vi "Add Correction.vi"(8 "error in (no error)":errorcluster, 9 "Assembly Type":string, 10 "XYZTheta":dbl[](array[numeric]), 11 "Carrier Tray in":refnum<class "Assembly Tray.lvclass">) -> (0 "error out":errorcluster, 2 "XYZTheta Out":dbl[](array[numeric]), 3 "Carrier Tray out":refnum<class "Assembly Tray.lvclass">)   [LabVIEW 2021, in "Assembly Tray.lvclass"]
uses:
  Assembly Tray.lvclass
  C:/Users/HEP/Documents/GitHub/Gantry/UCSB-Gantry-HEP-main/Classes/Workspace/Fixture.lvclass
  Fixture.lvclass/Fixture.ctl
  Read Fixture ID.vi
  Read Position.vi
  Routine/Pick and Place/Pick and Place.lvclass
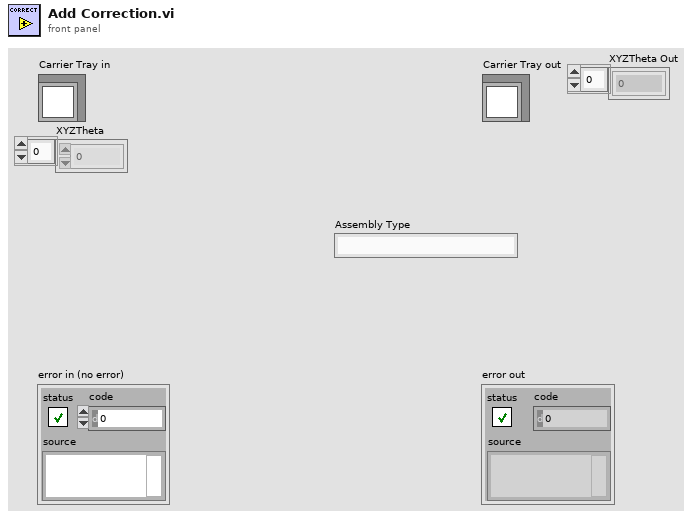
[diagram p1: front panel]
types:
  T1 = typedef "File Paths.ctl" = cluster{"Glue Pattern Folder":path, "Carrier Tray Folder":path, "Pick Up Tool Fixture Folder":path, "Components Folder":path, "Bellows Tool Offset.txt":path, "Pick Up Tool Offset.txt":path, "Dispense Tip Offset.txt":path, "Log Files":path, "Gantry Assembly Map.txt":path, "Syringe and offset map.txt":path, "Controllers Folder":path, "Local dbase config":path}
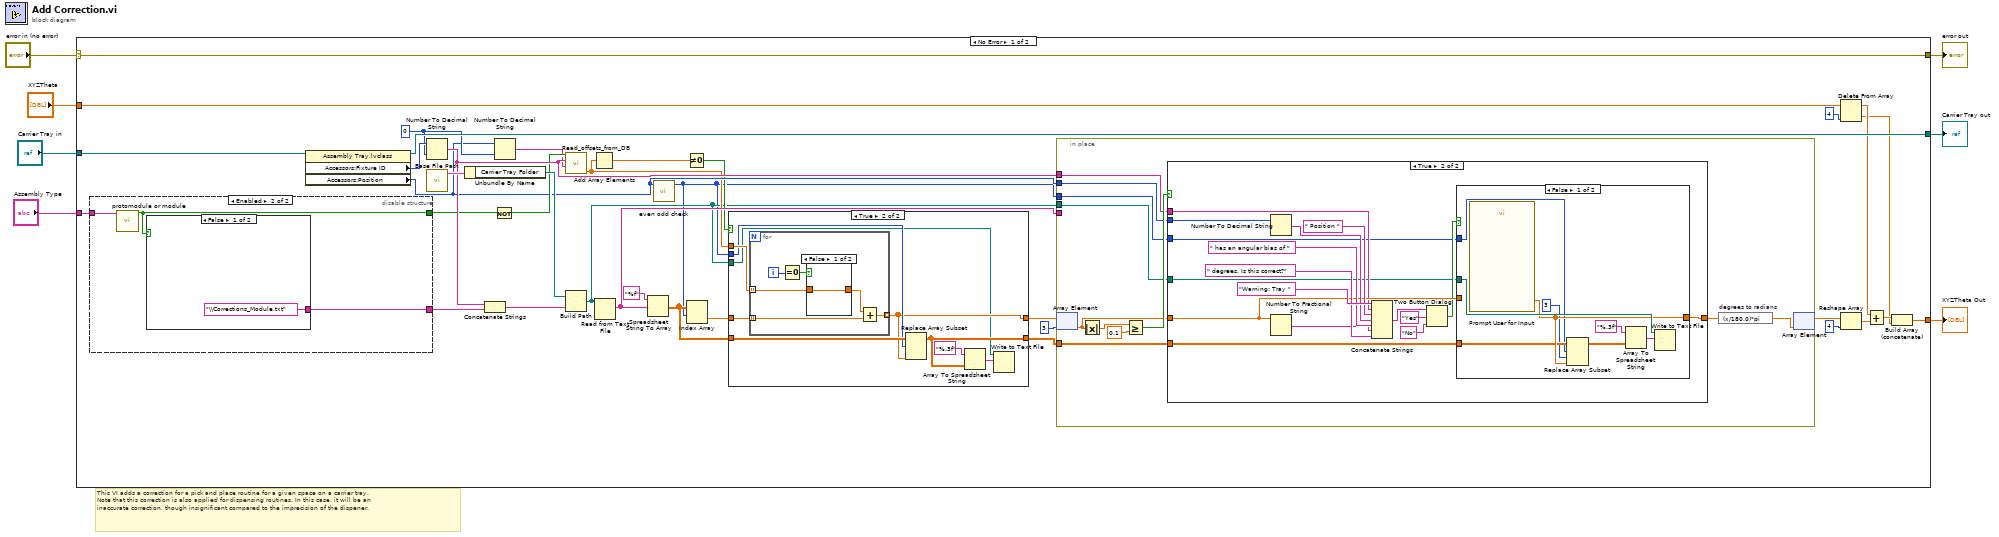
[diagram p0: block diagram]
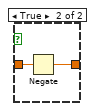
[diagram p3: hidden frame]
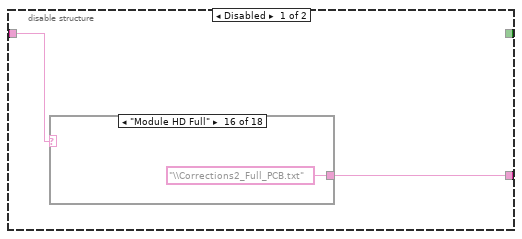
[diagram p6: hidden frame]
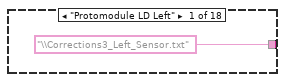
[diagram p7: hidden frame]
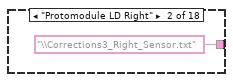
[diagram p8: hidden frame]
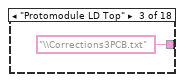
[diagram p9: hidden frame]
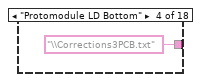
[diagram p10: hidden frame]
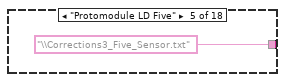
[diagram p11: hidden frame]
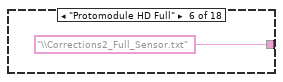
[diagram p12: hidden frame]
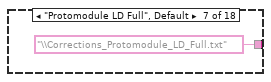
[diagram p13: hidden frame]
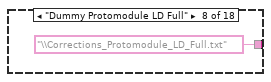
[diagram p14: hidden frame]
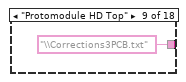
[diagram p15: hidden frame]
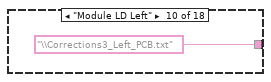
[diagram p16: hidden frame]
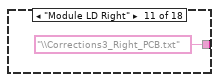
[diagram p17: hidden frame]
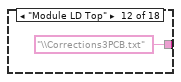
[diagram p18: hidden frame]
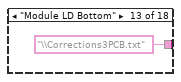
[diagram p19: hidden frame]
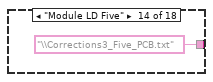
[diagram p20: hidden frame]
diagram:
  # "This VI adds a correction for a pick and place routine for a given space on a carrier tray.\nNote that this correction is also applied for dispensing routines. In this case, it will be an\ninaccurate correction, though insignificant compared to the imprecision of the dispener."
  n1 = case shown="No Error" "error in (no error)" {
    selector: "error in (no error)" -> [w43 w129]
    tunnel: [w43 w129] -> w6
    tunnel: [w34 w128] -> w4
    tunnel: "Carrier Tray in" -> [w35 w128]
    tunnel: "XYZTheta" -> [w31 w127]
    tunnel: [w26 w127] -> w2
    tunnel: "Assembly Type" -> [w32 _]
    frame No Error {
      w19 = i16 0 ("width (-)")
      n2 = disable-structure shown="Enabled" {
        disable-tunnel: [w103 w124] -> w40
        disable-tunnel: w32 -> [w102 w123]
        disable-tunnel: [_ w122] -> w21
        frame Disabled {
          n3 = case shown="\"Module HD Full\"" w102 {
            tunnel: ["\\Corrections3_Left_Sensor.txt" ("name or relative path") "\\Corrections3_Right_Sensor.txt" ("name or relative path") "\\Corrections3PCB.txt" ("name or relative path") "\\Corrections3PCB.txt" ("name or relative path") "\\Corrections3_Five_Sensor.txt" ("name or relative path") "\\Corrections2_Full_Sensor.txt" ("name or relative path") "\\Corrections_Protomodule_LD_Full.txt" ("name or relative path") "\\Corrections_Protomodule_LD_Full.txt" ("name or relative path") "\\Corrections3PCB.txt" ("name or relative path") "\\Corrections3_Left_PCB.txt" ("name or relative path") "\\Corrections3_Right_PCB.txt" ("name or relative path") "\\Corrections3PCB.txt" ("name or relative path") "\\Corrections3PCB.txt" ("name or relative path") "\\Corrections3_Five_PCB.txt" ("name or relative path") "\\Corrections2_Full_PCB.txt" ("name or relative path") "\\Corrections2_Full_PCB.txt" ("name or relative path") "\\Corrections_Module_LD_Full.txt" ("name or relative path") "\\Corrections_Module_LD_Full.txt" ("name or relative path")] -> w103
            frame "Protomodule LD Left" {
            }
            frame "Protomodule LD Right" {
            }
            frame "Protomodule LD Top" {
            }
            frame "Protomodule LD Bottom" {
            }
            frame "Protomodule LD Five" {
            }
            frame "Protomodule HD Full" {
            }
            frame "Protomodule LD Full", Default {
            }
            frame "Dummy Protomodule LD Full" {
            }
            frame "Protomodule HD Top" {
            }
            frame "Module LD Left" {
            }
            frame "Module LD Right" {
            }
            frame "Module LD Top" {
            }
            frame "Module LD Bottom" {
            }
            frame "Module LD Five" {
            }
            frame "Module HD Top" {
            }
            frame "Module HD Full" {
            }
            frame "Module LD Full" {
            }
            frame "Dummy Module LD Full" {
            }
          }
        }
        frame Enabled {
          n4 = call "protomodule or module.vi"("assembly type"=w123) -> ("protomodule? (T)"=w122:bool)  [unwired: 10 in]
          n5 = case shown="False" w122 {
            tunnel: ["\\Corrections_Module.txt" ("name or relative path") "\\Corrections_Protomodule.txt" ("name or relative path")] -> w124
            frame False {
            }
            frame True {
            }
          }
        }
      }
      n6 = property class="Assembly Tray.lvclass"(reference=w35) -> (reference out=w34:refnum<class "Assembly Tray.lvclass">, "Accessors:Fixture ID"=w33:i32, "Accessors:Position"=w18:i32)  [unwired: 1 in, 1 out]
      n7 = Number To Decimal String(number=w33, width (-)=w19) -> (decimal integer string=w22:string)
      n8 = call "Base File Path.vi"() -> ("Paths Out"=w42:T1)  [unwired: 11 in]
      n9 = Unbundle By Name(w42) -> ("Carrier Tray Folder"=w41:path)
      n10 = Concatenate Strings(w22, w40) -> (w39:string)
      n11 = Not(x=w21) -> (.not. x?=w20:bool)
      n12 = Number To Decimal String(number=w18, width (-)=w19) -> (decimal integer string=w17:string)
      n13 = call "Read_offsets_from_DB.vi"("PUT position"=w17, "Assembly Tray ID"=w22, "Module?"=w20) -> ("Bias to add"=w14:dbl[])  [unwired: 5 in, 3 out]
      n14 = Build Path(base path=w41, name or relative path=w39) -> (appended path=w11:path)
      n15 = Add Array Elements(numeric array=w14) -> (sum=w16:dbl)
      n16 = Read from Text File(file (use dialog)=w11) -> (text=w24:string)  [unwired: 3 in, 3 out]
      n17 = Spreadsheet String To Array(format string="%f", spreadsheet string=w24) -> (array=w10:dbl[][])  [unwired: 2 in]
      n18 = call "even odd check.vi"("position"=w18) -> ("index"=w8:i32)  [unwired: 10 in]
      n19 = Not Equal To 0?(x=w16) -> (x != 0?=w15:bool)
      n20 = Index Array(array=w10, index (row)=w8) -> (element=w13:dbl[])  [unwired: 1 in]
      n21 = case shown="True" w15 {
        tunnel: w14 -> [_ w54]
        tunnel: w13 -> [w45 w53]
        tunnel: [w45 w50] -> w12
        tunnel: w11 -> [_ w46]
        tunnel: w10 -> [w44 w52]
        tunnel: [w44 w47] -> w9
        tunnel: w8 -> [_ w51]
        frame False {
        }
        frame True {
          n22 = for {
            tunnel: w54 -> [w58] mode=indexing
            tunnel: w53 -> [w56] mode=indexing
            tunnel: [w55] -> w50 mode=indexing
            i -> [w60]
            n23 = Equal To 0?(x=w60) -> (x = 0?=w59:bool)
            n24 = case shown="False" w59 {
              tunnel: w58 -> [w61 w63]
              tunnel: [w61 w62] -> w57
              frame False {
              }
              frame True {
                n25 = Negate(x=w63) -> (-x=w62:dbl)
              }
            }
            n26 = Add(x=w57, y=w56) -> (x+y=w55:dbl)
          }
          n27 = Replace Array Subset(array=w52, new element=w50, index (row)=w51) -> (w47:dbl[][])  [unwired: 1 in]
          n28 = Array To Spreadsheet String(array=w47, 3:"%.3f" ("format string")) -> (spreadsheet string=w49:string)  [unwired: 1 in]
          n29 = Write to Text File(file (use dialog)=w46, text=w49) -> ()  [unwired: 2 in, 3 out]
        }
      }
      n30 = in-place {
        in-place-border: w24 -> [_]
        in-place-border: w18 -> [w69]
        in-place-border: w22 -> [w67]
        in-place-border: w11 -> [w66]
        in-place-border: w9 -> [w65]
        in-place-border: w8 -> [w64]
        n31 = in-place-array #1(w12, 3) -> (w68:dbl)
        n32 = Absolute Value(x=w68) -> (abs(x)=w73:dbl)
        n33 = Greater Or Equal?(x=w73, y=0.1) -> (x >= y?=w71:bool)
        n34 = case shown="True" w71 {
          tunnel: [w75 w84] -> w70
          tunnel: w69 -> [_ w89]
          tunnel: w68 -> [w75 w83]
          tunnel: w67 -> [_ w80]
          tunnel: w66 -> [_ w78]
          tunnel: w65 -> [_ w77]
          tunnel: w64 -> [_ w76]
          frame False {
          }
          frame True {
            n35 = Number To Decimal String(number=w89) -> (decimal integer string=w88:string)  [unwired: 1 in]
            n36 = Number To Fractional String(number=w83) -> (F-format string=w85:string)  [unwired: 3 in]
            n37 = Concatenate Strings("Warning: Tray " ("string"), w80, " Position " ("string"), w88, " has an angular bias of " ("string"), w85, " degrees. Is this correct?" ("string")) -> (w92:string)
            n38 = Two Button Dialog(message=w92, 1:"No" ("F button name (\"Cancel\")"), 2:"Yes" ("T button name (\"OK\")")) -> (T button?=w79:bool)
            n39 = case shown="False" w79 {
              tunnel: [w97 w101] -> w84
              tunnel: w83 -> [_ w101]
              tunnel: w78 -> [w98 _]
              tunnel: w77 -> [w96 _]
              tunnel: w76 -> [w95 _]
              frame False {
                n40 = call "Prompt User for Input"() -> ("angle_bias"=w97:dbl)  [unwired: 17 in, 2 out]
                n41 = Replace Array Subset(array=w96, new element=w97, index (row)=w95, index (col)=3 ("disabled index (col)")) -> (w93:dbl[][])
                n42 = Array To Spreadsheet String(array=w93, 3:"%.3f" ("format string")) -> (spreadsheet string=w100:string)  [unwired: 1 in]
                n43 = Write to Text File(file (use dialog)=w98, text=w100) -> ()  [unwired: 2 in, 3 out]
              }
              frame True {
              }
            }
          }
        }
        n44 = expression code="(x/180.0)*pi" "degrees to radians"(w70) -> (w74:dbl)
        n45 = in-place-array #1(w74) -> (w23:dbl[])  [unwired: 1 out]
      }
      n46 = Delete From Array(array=w31, index=4) -> (deleted portion=w27:dbl, array with subset deleted=w29:dbl[])  [unwired: 1 in]
      n47 = Reshape Array(w23, 4 ("dimension size")) -> (w36:dbl[])
      n48 = Add(x=w29, y=w36) -> (x+y=w28:dbl[])
      n49 = Build Array (concatenate)(w28, w27) -> (w26:dbl[])
    }
    frame Error {
    }
  }
  "error out" <- w6
  "Carrier Tray out" <- w4
  "XYZTheta Out" <- w2
